vi "ionization_average.vi"() -> ()   [LabVIEW 2016]
uses:
  <instrlib>/tektronix_7000_series/Tektronix 7000 Series/Public/Data/Read (Single Waveform).vi
  <instrlib>/tektronix_7000_series/Tektronix 7000 Series/Tektronix 7000 Series.lvlib
panel:
  out "Oscilloscope Reading":waveform(dbl)(graph)={"t0"=timestamp(5.451199999967175e-09 s since 1904-01-01), "dt"=8e-09, "Y"=[0.06, 0.1, 0.06, 0.1, 0.08, 0.1, 0.1, 0.1, 0.04, 0.06, 0.12, 0.1, 0.1, 0.08, 0.08, 0.08, 0.06, 0.1, 0.12, 0.06, 0.06, 0.06, 0.06, -0.02, 0.08, 0.06, 0.08, 0.1, 0.1, 0.1, 0.08, 0.08, 0.08, 0.1, 0.12, 0.06, 0.08, 0.08, 0.06, 0.08, 0.08, 0.08, 0.12, 0.08, 0.06, 0.06, 0.1, 0.06, 0.08, 0.1, 0.08, 0.1, 0.08, 0.06, 0.12, 0.1, 0.1, 0.08, 0.08, 0.08, 0.1, 0.08, 0.1, 0.08, 0.1, 0.08, 0.1, 0.06, 0.1, 0.04, 0.06, 0.12, 0.08, 0.14, 0.1, 0.12, 0.1, 0.1, 0.06, 0.12, 0.08, 0.12, 0.14, 0.06, 0.06, 0.12, 0.08, 0.08, 0.12, 0.06, 0.08, 0.1, 0.1, 0.12, 0.1, 0.06, 0.12, 0.06, 0.08, 0.04, 0.12, 0.06, 0.08, 0.08, 0.08, 0.04, 0.1, 0.08, 0.1, 0.06, 0.06, 0.08, 0.1, 0.08, 0.1, 0.06, 0.12, 0.06, 0.1, 0.08, 0.1, 0.1, 0.08, 0.1, 0.1, 0.1, 0.08, 0.08, 0.1, 0.06, 0.1, 0.06, 0.1, 0.08, 0.08, 0.1, 0.1, 0.08, 0.1, 0.08, 0.08, 0.06, 0.08, 0.08, 0.14, 0.08, 0.06, 0.1, 0.1, 0.08, 0.12, 0.12, 0.1, 0.06, 0.1, 0.1, 0.12, 0.06, 0.1, 0.1, 0.1, 0.06, 0.1, 0.12, 0.12, 0.08, 0.08, 0.08, 0.12, 0.08, 0.1, 0.08, 0.1, 0.16, 0.16, -0.04, 0.21999999999999997, 0.04, 0.08, 0.08, 0.1, 0.06, 0.1, 0.08, 0.1, 0.04, 0.08, 0.06, 0.08, 0.04, 0.08, 0.1, 0.12, 0.06, 0.08, 0.06, 0.08, 0.1, 0.12, 0.06, 0.12, 0.06, 0.08, 0.06, 0.06, 0.06, 0.12, 0.1, 0.08, 0.06, 0.1, 0.04, 0.1, 0.06, 0.08, 0.08, 0.1, 0.04, 0.1, 0.04, 0.08, 0.08, 0.08, -0.02, 0.06, 0.0, 0.14, 0.04, 0.1, 0.04, 0.1, 0.08, 0.1, 0.06, 0.06, 0.1, 0.1, 0.08, 0.08, 0.06, 0.1, 0.06, 0.1, 0.08, 0.1, 0.08, 0.08, 0.1, 0.1, 0.1, 0.1, 0.08, 0.1, 0.06, 0.1, 0.1, 0.1, 0.06, 0.1, 0.1, 0.12, 0.08, 0.08, 0.12, 0.08, 0.06, 0.1, 0.12, 0.06, 0.06, 0.1, 0.1, 0.1, 0.06, 0.08, 0.1, 0.06, 0.06, 0.06, 0.1, 0.08, 0.06, 0.06, 0.12, 0.06, 0.08, 0.1, 0.06, 0.06, 0.06, 0.1, 0.1, 0.08, 0.14, 0.08, 0.1, 0.06, 0.08, 0.1, 0.08, 0.1, 0.06, 0.12, 0.06, 0.04, 0.12, 0.08, 0.1, 0.08, 0.08, 0.08, 0.1, 0.06, 0.08, 0.08, 0.06, 0.08, 0.08, 0.1, 0.1, 0.08, 0.08, 0.06, 0.08, 0.06, 0.08, 0.12, 0.06, 0.06, 0.06, 0.08, 0.1, 0.08, 0.08, 0.12, 0.08, 0.08, 0.1, 0.08, 0.1, 0.1, 0.1, 0.12, 0.08, 0.1, 0.1, 0.08, 0.1, 0.06, 0.08, 0.1, 0.08, 0.06, 0.1, 0.06, 0.08, 0.1, 0.08, 0.06, 0.08, 0.06, 0.08, 0.06, 0.08, 0.08, 0.08, 0.04, 0.1, 0.1, 0.12, 0.08, 0.12, 0.06, 0.18000000000000002, 0.02, 0.0, 0.12, 0.04, 0.08, 0.08, 0.04, 0.08, 0.06, 0.04, 0.08, 0.08, 0.06, 0.1, 0.12, 0.04, 0.08, 0.08, 0.06, 0.12, 0.06, 0.06, 0.08, 0.06, 0.08, 0.12, 0.08, 0.08, 0.02, 0.04, 0.04, 0.1, 0.08, 0.08, 0.04, 0.1, 0.06, 0.08, 0.04, 0.1, 0.06, 0.08, 0.08, 0.08, 0.06, 0.06, 0.08, 0.12, 0.04, 0.0, 0.08, 0.06, 0.08, 0.12, 0.1, 0.08, 0.1, 0.08, 0.08, 0.1, 0.04, 0.1, 0.06, 0.08, 0.1, 0.1, 0.06, 0.12, 0.06, 0.1, 0.1, 0.06, 0.08, 0.08, 0.08, 0.1, 0.06, 0.1, 0.1, 0.12, 0.02, 0.12, 0.08, 0.12, 0.06, 0.08, 0.1, 0.1, 0.06, 0.08, 0.08, 0.1, 0.06, 0.1, 0.06, 0.12, 0.08, 0.12, 0.1, 0.08, 0.08, 0.1, 0.08, 0.1, 0.08, 0.08, 0.12, 0.12, 0.08, 0.14, 0.08, 0.08, 0.08, 0.08, 0.1, 0.12, 0.08, 0.1, 0.1, 0.12, 0.06, 0.1, 0.06, 0.12, 0.06, 0.1]}
  in  "Maximum Time (10000 ms)":u32=100000000
  in  "Probe Attenuation (10.0)":dbl=10.0
  in  "Channel (0: Channel 1)":u16(ring) format="%#_5f" items=["Channel 1", "Channel 2", "Channel 3", "Channel 4"]
  in  "VISA Resource Name":refnum<visa-resource-name>="tds5052b"
  in  "Average #":i32=5
  out "0.5*Max intens":dbl=0.06999999999999998
  in  "Final Position, mm":ext=8.6625000000000000003
  out "Pulse":dbl[][](graph)
  in  "Start FROG":bool
  in  "Initial Position, mm":ext=8.6618999999999999996
  in  "Step Size, mm":ext=0.0001
  in  "MG17Motor":refnum<k7>(container)
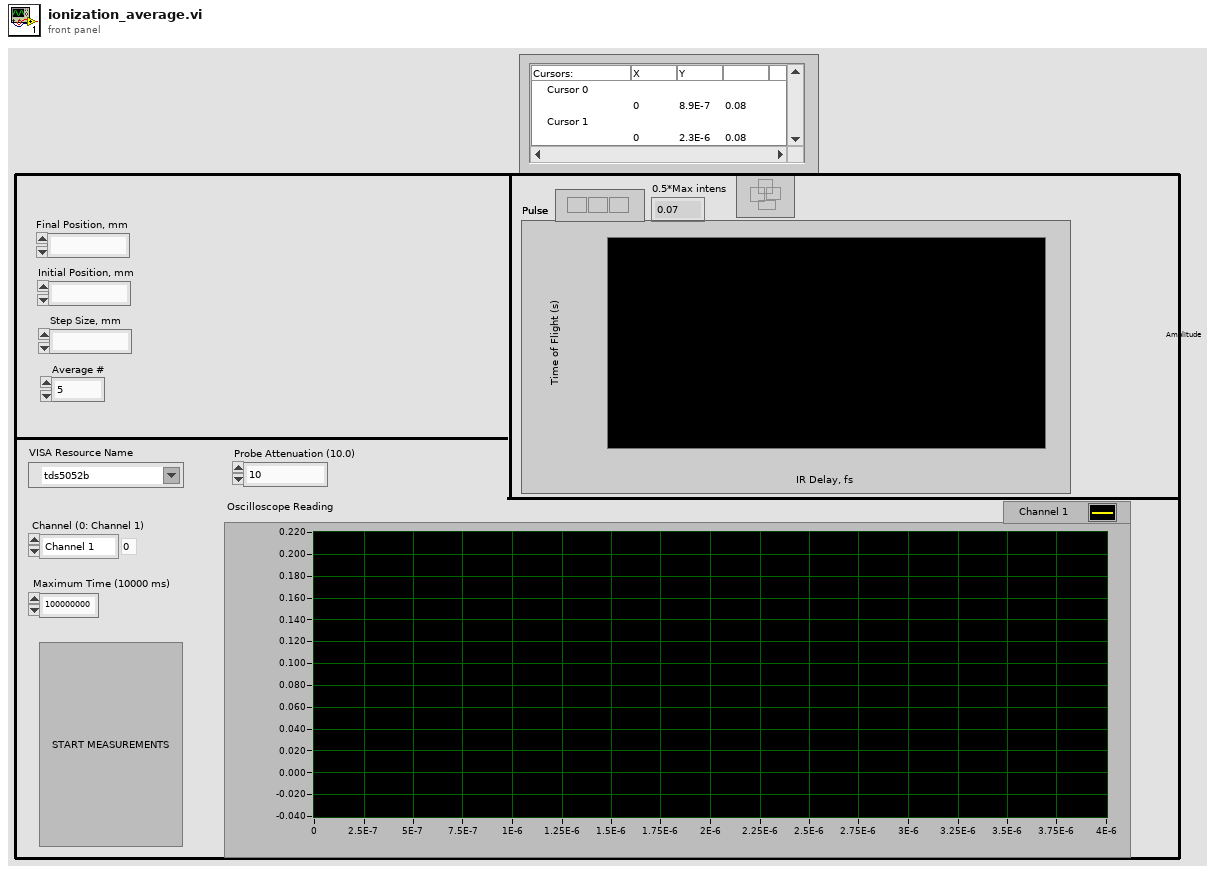
[diagram p1: front panel]
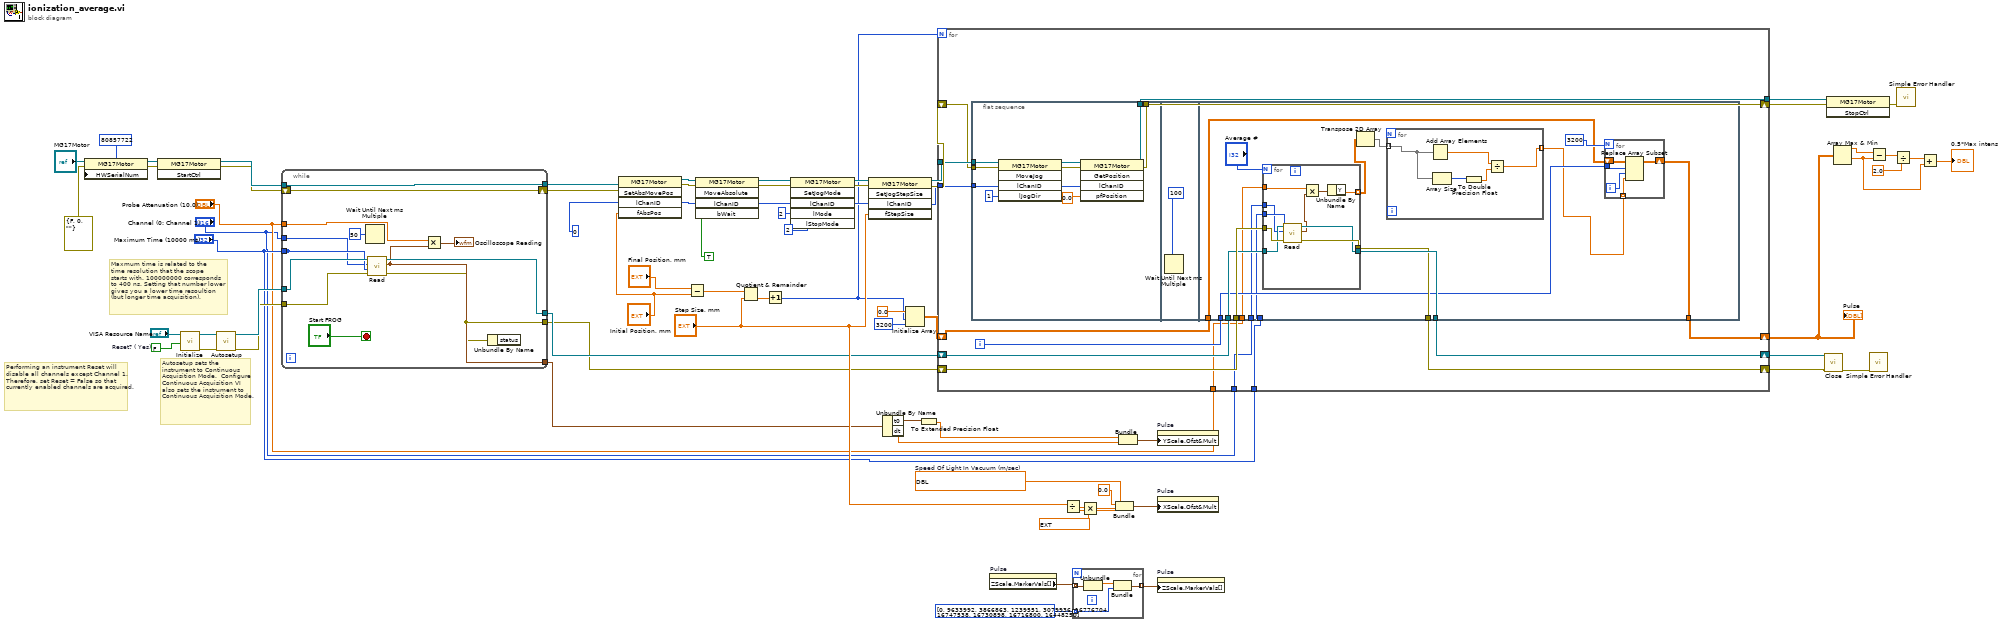
[diagram p0: block diagram]
diagram:
  w17 = FALSE  # Reset? ( Yes)
  w71 = ext[unit] 299792458.0  # Speed Of Light In Vacuum (m/sec)
  # "Maxmum time is related to the\ntime resolution that the scope\nstarts with. 100000000 corresponds\nto 400 ns. Setting that number lower\ngives you a lower time resoultion \n(but longer time acquisition)."
  # "Autosetup sets the instrument to Continuous Acquisition Mode.  Configure Continuous Acquisition VI also sets the instrument to Continuous Acquisition Mode."
  # "Performing an instrument Reset will disable all channels except Channel 1. Therefore, set Reset = False so that currently enabled channels are acquired."
  n1 = property class="MG17Motor"(reference="MG17Motor", error in=errorcluster {"status"=FALSE, "code"=0, "source"=""} ("error in (no error)"), "HWSerialNum"=80857722) -> (reference out=w59:refnum<k7>, error out=w58:errorcluster)
  n2 = invoke class="MG17Motor" method="StartCtrl"(reference=w59, error in=w58) -> (reference out=w39:refnum<k7>, error out=w38:errorcluster)  [unwired: 1 in, 1 out]
  n3 = call <instrlib>:"Initialize.vi"("Reset? ( Yes)"=w17, "VISA resource name"="VISA Resource Name") -> ("error out"=w15:errorcluster, "VISA resource name out"=w16:refnum<visa-resource-name>)  [unwired: 8 in]
  n4 = call <instrlib>:"Autosetup.vi"("error in (no error)"=w15, "VISA resource name"=w16) -> ("error out"=w13:errorcluster, "VISA resource name out"=w14:refnum<visa-resource-name>)  [unwired: 8 in]
  n5 = while {
    tunnel: w39 -> [w84]
    tunnel: [w84] -> w21
    shift-right: [w83] -> w20
    shift-left: w38 -> [w83]
    tunnel: w14 -> [w78]
    tunnel: w13 -> [w77]
    tunnel: "Probe Attenuation (10.0)" -> [w80]
    tunnel: "Channel (0: Channel 1)" -> [w75]
    tunnel: [w76] -> _
    tunnel: "Maximum Time (10000 ms)" -> [w76]
    tunnel: [w79] -> w8
    tunnel: [w73] -> w7
    tunnel: [w74] -> w12
    stop <- "Start FROG" stop-if-true
    n6 = Wait Until Next ms Multiple(millisecond multiple=u32 50) -> ()  [unwired: 1 out]
    n7 = call-poly <instrlib>:"Read.vi"("error in (no error)"=w77, "Maximum Time (10000 ms)"=w76, "Channel (0: Channel 1)"=w75, "VISA resource name"=w78) -> ("error out"=w73:errorcluster, "Waveform Data"=w74:waveform(dbl), "VISA resource name out"=w79:refnum<visa-resource-name>)  [unwired: 5 in]
    n8 = Multiply(x=w80, y=w74) -> (x*y=→"Oscilloscope Reading":waveform(dbl))
    n9 = Unbundle By Name(w73) -> ()  [unwired: 1 out]
  }
  n10 = invoke class="MG17Motor" method="SetAbsMovePos"(reference=w21, error in=w20, "lChanID"=0, "fAbsPos"="Initial Position, mm") -> (reference out=w51:refnum<k7>, error out=w50:errorcluster, "lChanID"=w48:i32)  [unwired: 1 in, 2 out]
  n11 = Subtract(x="Final Position, mm", y="Initial Position, mm") -> (x-y=w34:ext)
  n12 = invoke class="MG17Motor" method="MoveAbsolute"(reference=w51, error in=w50, "lChanID"=w48, "bWait"=TRUE) -> (reference out=w42:refnum<k7>, error out=w41:errorcluster, "lChanID"=w47:i32)  [unwired: 1 in, 2 out]
  n13 = Quotient & Remainder(x=w34, y="Step Size, mm") -> (floor(x/y)=w33:ext)  [unwired: 1 out]
  n14 = Increment(x=w33) -> (x+1=w30:i32)
  n15 = invoke class="MG17Motor" method="SetJogMode"(reference=w42, error in=w41, "lChanID"=w47, "lMode"=2, "lStopMode"=2) -> (reference out=w56:refnum<k7>, error out=w54:errorcluster, "lChanID"=w46:i32)  [unwired: 1 in, 3 out]
  n16 = invoke class="MG17Motor" method="SetJogStepSize"(reference=w56, error in=w54, "lChanID"=w46, "fStepSize"="Step Size, mm") -> (reference out=w55:refnum<k7>, error out=w53:errorcluster, "lChanID"=w45:i32)  [unwired: 1 in, 2 out]
  n17 = Unbundle By Name(w12) -> ("t0"=w10:timestamp, "dt"=w11:dbl)
  n18 = Initialize Array(0.0 ("element"), w30, 3200 ("dimension size")) -> (w29:dbl[][])
  n19 = To Extended Precision Float(1:w10) -> (0:w9:ext)
  n20 = for {
    N: w30 -> [_]
    tunnel: w55 -> [w100]
    tunnel: [w95] -> w37
    tunnel: w45 -> [w98]
    shift-right: [w93] -> w2
    shift-left: w8 -> [w97]
    shift-right: [w92] -> w1
    shift-left: w7 -> [w96]
    shift-right: [w89] -> w28
    shift-left: w29 -> [w91]
    shift-right: [w94] -> w49
    shift-left: w53 -> [w99]
    tunnel: "Maximum Time (10000 ms)" -> [w86]
    tunnel: "Probe Attenuation (10.0)" -> [w88]
    tunnel: "Channel (0: Channel 1)" -> [w87]
    i -> [w90]
    n21 = flat-sequence {
      tunnel: w100 -> [w105]
      tunnel: w99 -> [w104]
      tunnel: w98 -> [w103]
      tunnel: [w101] -> w95
      tunnel: [w102] -> w94
      tunnel: w97 -> [w122]
      tunnel: w96 -> [w123]
      tunnel: [w120] -> w92
      tunnel: [w121] -> w93
      tunnel: w90 -> [w119]
      tunnel: w91 -> [w125]
      tunnel: [w124] -> w89
      tunnel: w88 -> [w115]
      tunnel: w87 -> [w114]
      tunnel: w86 -> [w113]
      frame #0 {
        n22 = invoke class="MG17Motor" method="MoveJog"(reference=w105, error in=w104, "lChanID"=w103, "lJogDir"=1) -> (reference out=w109:refnum<k7>, error out=w110:errorcluster, "lChanID"=w106:i32)  [unwired: 1 in, 2 out]
        n23 = invoke class="MG17Motor" method="GetPosition"(reference=w109, error in=w110, "lChanID"=w106, "pfPosition"=sgl 0.0) -> (reference out=w101:refnum<k7>, error out=w102:errorcluster)  [unwired: 1 in, 3 out]
      }
      frame #1 {
        n24 = Wait Until Next ms Multiple(millisecond multiple=u32 100) -> ()  [unwired: 1 out]
      }
      frame #2 {
        n25 = for {
          N: "Average #" -> [_]
          tunnel: [w141] -> w117 mode=indexing
          tunnel: w123 -> [w138]
          tunnel: [w140] -> w120
          tunnel: w122 -> [w137]
          tunnel: [w139] -> w121
          tunnel: w115 -> [w133]
          tunnel: w114 -> [w135]
          tunnel: w113 -> [w136]
          n26 = call-poly <instrlib>:"Read.vi"("error in (no error)"=w138, "Maximum Time (10000 ms)"=w136, "Channel (0: Channel 1)"=w135, "VISA resource name"=w137) -> ("error out"=w140:errorcluster, "Waveform Data"=w134:waveform(dbl), "VISA resource name out"=w139:refnum<visa-resource-name>)  [unwired: 5 in]
          n27 = Multiply(x=w133, y=w134) -> (x*y=w132:waveform(dbl))
          n28 = Unbundle By Name(w132) -> ("Y"=w141:dbl[])
        }
        n29 = Transpose 2D Array(2D array=w117) -> (transposed array=w116:dbl[][])
        n30 = for {
          tunnel: [w128] -> w112 mode=indexing
          tunnel: w116 -> [w127] mode=indexing
          n31 = Add Array Elements(numeric array=w127) -> (sum=w129:dbl)
          n32 = Array Size(array=w127) -> (size(s)=w131:i32)
          n33 = To Double Precision Float(number=w131) -> (double precision float=w130:dbl)
          n34 = Divide(x=w129, y=w130) -> (x/y=w128:dbl)
        }
        n35 = for {
          N: 3200 -> [_]
          shift-right: [w145] -> w124
          shift-left: w125 -> [w146]
          tunnel: w119 -> [w142]
          tunnel: w112 -> [w144] mode=indexing
          i -> [w143]
          n36 = Replace Array Subset(array=w146, new element=w144, index (row)=w142, index (col)=w143) -> (w145:dbl[][])
        }
      }
    }
  }
  "Pulse" <- w28
  n37 = property on="Pulse" class="IntGraph (strict)"() -> ("ZScale.MarkerVals[]"=w64:cluster{dbl, u32}[])  [unwired: 2 in, 2 out]
  n38 = Divide(x="Step Size, mm", y=w71) -> (x/y=w70:ext)
  n39 = for {
    tunnel: w64 -> [w150] mode=indexing
    tunnel: u32[] [0, 9633992, 3866863, 1239551, 3079936, 16776704, 16747538, 16730898, 16716800, 16448250] ("Custom Marker Colors 2") -> [w148] mode=indexing
    tunnel: [w147] -> w63 mode=indexing
    n40 = Unbundle(w150) -> (w149:dbl)  [unwired: 1 out]
    n41 = Bundle(w149, "Color Box"=w148) -> (w147:cluster{dbl, "Color Box":u32})  [unwired: 1 in]
  }
  n42 = Multiply(x=w70, y=ext 2000000000000.0) -> (x*y=w66:ext)
  n43 = Bundle(0.0, w66) -> (w67:cluster{dbl, ext})  [unwired: 1 in]
  n44 = Bundle(w9, "dt"=w11) -> (w72:cluster{ext, "dt":dbl})  [unwired: 1 in]
  n45 = property on="Pulse" class="IntGraph (strict)"("YScale.Ofst&Mult"=w72) -> ()  [unwired: 2 in, 2 out]
  n46 = property on="Pulse" class="IntGraph (strict)"("XScale.Ofst&Mult"=w67) -> ()  [unwired: 2 in, 2 out]
  n47 = property on="Pulse" class="IntGraph (strict)"("ZScale.MarkerVals[]"=w63) -> ()  [unwired: 2 in, 2 out]
  n48 = call <instrlib>:"Close.vi"("error in (no error)"=w1, "VISA resource name"=w2) -> ("error out"=w3:errorcluster)  [unwired: 9 in]
  n49 = invoke class="MG17Motor" method="StopCtrl"(reference=w37, error in=w49) -> (error out=w40:errorcluster)  [unwired: 1 in, 2 out]
  n50 = Array Max & Min(array=w28) -> (max value=w27:dbl, min value=w23:dbl)  [unwired: 2 out]
  n51 = call <vilib>:"Simple Error Handler.vi"("error in (no error)"=w3) -> ()  [unwired: 1 in, 8 out]
  n52 = Subtract(x=w27, y=w23) -> (x-y=w26:dbl)
  n53 = Divide(x=w26, y=2.0) -> (x/y=w24:dbl)
  n54 = call <vilib>:"Simple Error Handler.vi"("error in (no error)"=w40) -> ()  [unwired: 1 in, 8 out]
  n55 = Add(x=w24, y=w23) -> (x+y=→"0.5*Max intens":dbl)
